vi "HandleObservationSync.vi"(8 "error in (no error)":errorcluster, 11 "S4GUI in":refnum<class "S4GUI.lvclass">) -> (0 "error out":errorcluster, 3 "S4GUI out":refnum<class "S4GUI.lvclass">)   [LabVIEW 2018, in "S4GUI.lvclass"] (continued)
          n1278 = call-dynamic "VerifyAcqIdle.vi"("error in (no error)"=w3499, "S4GUI in"=w3498) -> ("error out"=w3504:errorcluster, "idle"=w3503:bool, "S4GUI out"=w3505:refnum<class "S4GUI.lvclass">)  [unwired: 6 in, 1 out]
          n1279 = disable-structure shown="Enabled" {
            disable-tunnel: w3501 -> [w3508 _]
            disable-tunnel: [w3507 u32 325] -> w3500
            frame Disabled {
              n1280 = Increment(x=w3508) -> (x+1=w3507:u32)
            }
            frame Enabled {
            }
          }
          n1281 = Select(t=w3500, s=w3503, f=w3501) -> (s? t:f=w3502:u32)
          n1282 = Bundle By Name(cluster=w3505, "Obs_state"=w3502) -> (w3506:refnum<class "S4GUI.lvclass">)
        }
        frame 323 {
          n1283 = call-dynamic "Read AcquisitionA.vi"("error in (no error)"=w3572, "S4ACS_GUI in"=w3573) -> ("error out"=w3527:errorcluster, "Acquisition.lvclass"=w3528:refnum<class "Acquisition.lvclass">, "S4ACS_GUI out"=w3575:refnum<class "S4GUI.lvclass">)  [unwired: 7 in]
          n1284 = call-dynamic "Read enabled.vi"("error in (no error)"=w3527, "Server in"=w3528) -> ("error out"=w3526:errorcluster, "enabled"=w3513:bool, "Server out"=w3529:refnum<class "Acquisition.lvclass">)  [unwired: 7 in]
          n1285 = call "Read connection.vi"("error in (no error)"=w3526, "Server in"=w3529) -> ("error out"=w3552:errorcluster, "connection"=w3536:bool, "Server out"=w3553:refnum<class "Acquisition.lvclass">)  [unwired: 7 in]
          n1286 = And(x=w3536, y=w3513) -> (x .and. y?=w3537:bool)
          n1287 = case shown="True" w3537 {
            tunnel: w3553 -> [w3682 w3698]
            tunnel: w3552 -> [w3681 w3697]
            tunnel: [w3682 w3695] -> w3576
            tunnel: [w3681 w3694] -> w3574
            tunnel: [w3678 u32 0 ("New_State")] -> w3542
            tunnel: w3513 -> [w3677 _]
            frame False {
              n1288 = Select(t=u32 1, s=w3677, f=u32 0) -> (s? t:f=w3678:u32)
            }
            frame True {
              n1289 = call-dynamic "Read Channel.vi"("error in (no error)"=w3697, "Acquisition in"=w3698) -> ("error out"=w3690:errorcluster, "Channel.lvclass"=w3689:refnum<class "Channel.lvclass">, "Acquisition out"=w3696:refnum<class "Acquisition.lvclass">)  [unwired: 7 in]
              n1290 = call-dynamic "Read State Machine.vi"("error in (no error)"=w3690, "Device in"=w3689) -> ("error out"=w3691:errorcluster, "State Machine.lvclass"=w3693:refnum<class "State Machine.lvclass">, "Device out"=w3687:refnum<class "Channel.lvclass">)  [unwired: 7 in]
              n1291 = call "Next State.vi"("error in (no error)"=w3691, "New_State"=50, "State Machine in"=w3693) -> ("error out"=w3684:errorcluster, "State Machine out"=w3685:refnum<class "State Machine.lvclass">)  [unwired: 7 in]
              n1292 = call-dynamic "Write State Machine.vi"("error in (no error)"=w3684, "State Machine.lvclass"=w3685, "Device in"=w3687) -> ("error out"=w3686:errorcluster, "Device out"=w3688:refnum<class "Channel.lvclass">)  [unwired: 7 in]
              n1293 = call-dynamic "Write Channel.vi"("error in (no error)"=w3686, "Channel.lvclass"=w3688, "Acquisition in"=w3696) -> ("error out"=w3694:errorcluster, "Acquisition out"=w3695:refnum<class "Acquisition.lvclass">)  [unwired: 7 in]
            }
          }
          n1294 = call-dynamic "Write AcquisitionA.vi"("error in (no error)"=w3574, "Acquisition.lvclass"=w3576, "S4ACS_GUI in"=w3575) -> ("error out"=w3569:errorcluster, "S4ACS_GUI out"=w3570:refnum<class "S4GUI.lvclass">)  [unwired: 7 in]
          n1295 = call "Read AcquisitionB.vi"("error in (no error)"=w3569, "S4ACS_GUI in"=w3570) -> ("error out"=w3523:errorcluster, "Acquisition.lvclass"=w3525:refnum<class "Acquisition.lvclass">, "S4ACS_GUI out"=w3567:refnum<class "S4GUI.lvclass">)  [unwired: 7 in]
          n1296 = call-dynamic "Read enabled.vi"("error in (no error)"=w3523, "Server in"=w3525) -> ("error out"=w3522:errorcluster, "enabled"=w3512:bool, "Server out"=w3524:refnum<class "Acquisition.lvclass">)  [unwired: 7 in]
          n1297 = call "Read connection.vi"("error in (no error)"=w3522, "Server in"=w3524) -> ("error out"=w3550:errorcluster, "connection"=w3534:bool, "Server out"=w3551:refnum<class "Acquisition.lvclass">)  [unwired: 7 in]
          n1298 = And(x=w3534, y=w3512) -> (x .and. y?=w3535:bool)
          n1299 = case shown="True" w3535 {
            tunnel: w3551 -> [w3660 w3676]
            tunnel: w3550 -> [w3659 w3675]
            tunnel: [w3660 w3673] -> w3568
            tunnel: [w3659 w3672] -> w3566
            tunnel: [w3656 u32 0 ("New_State")] -> w3541
            tunnel: w3512 -> [w3655 _]
            frame False {
              n1300 = Select(t=u32 2, s=w3655, f=u32 0) -> (s? t:f=w3656:u32)
            }
            frame True {
              n1301 = call-dynamic "Read Channel.vi"("error in (no error)"=w3675, "Acquisition in"=w3676) -> ("error out"=w3668:errorcluster, "Channel.lvclass"=w3667:refnum<class "Channel.lvclass">, "Acquisition out"=w3674:refnum<class "Acquisition.lvclass">)  [unwired: 7 in]
              n1302 = call-dynamic "Read State Machine.vi"("error in (no error)"=w3668, "Device in"=w3667) -> ("error out"=w3669:errorcluster, "State Machine.lvclass"=w3671:refnum<class "State Machine.lvclass">, "Device out"=w3665:refnum<class "Channel.lvclass">)  [unwired: 7 in]
              n1303 = call "Next State.vi"("error in (no error)"=w3669, "New_State"=50, "State Machine in"=w3671) -> ("error out"=w3662:errorcluster, "State Machine out"=w3663:refnum<class "State Machine.lvclass">)  [unwired: 7 in]
              n1304 = call-dynamic "Write State Machine.vi"("error in (no error)"=w3662, "State Machine.lvclass"=w3663, "Device in"=w3665) -> ("error out"=w3664:errorcluster, "Device out"=w3666:refnum<class "Channel.lvclass">)  [unwired: 7 in]
              n1305 = call-dynamic "Write Channel.vi"("error in (no error)"=w3664, "Channel.lvclass"=w3666, "Acquisition in"=w3674) -> ("error out"=w3672:errorcluster, "Acquisition out"=w3673:refnum<class "Acquisition.lvclass">)  [unwired: 7 in]
            }
          }
          n1306 = call "Write AcquisitionB.vi"("error in (no error)"=w3566, "Acquisition.lvclass"=w3568, "S4ACS_GUI in"=w3567) -> ("error out"=w3562:errorcluster, "S4ACS_GUI out"=w3561:refnum<class "S4GUI.lvclass">)  [unwired: 7 in]
          n1307 = call-dynamic "Read AcquisitionC.vi"("error in (no error)"=w3562, "S4ACS_GUI in"=w3561) -> ("error out"=w3519:errorcluster, "Acquisition.lvclass"=w3521:refnum<class "Acquisition.lvclass">, "S4ACS_GUI out"=w3564:refnum<class "S4GUI.lvclass">)  [unwired: 7 in]
          n1308 = call-dynamic "Read enabled.vi"("error in (no error)"=w3519, "Server in"=w3521) -> ("error out"=w3518:errorcluster, "enabled"=w3511:bool, "Server out"=w3520:refnum<class "Acquisition.lvclass">)  [unwired: 7 in]
          n1309 = call "Read connection.vi"("error in (no error)"=w3518, "Server in"=w3520) -> ("error out"=w3548:errorcluster, "connection"=w3531:bool, "Server out"=w3549:refnum<class "Acquisition.lvclass">)  [unwired: 7 in]
          n1310 = And(x=w3531, y=w3511) -> (x .and. y?=w3533:bool)
          n1311 = case shown="True" w3533 {
            tunnel: [w3637 w3646] -> w3565
            tunnel: [w3638 w3645] -> w3563
            tunnel: w3549 -> [w3638 w3643]
            tunnel: w3548 -> [w3637 w3642]
            tunnel: [w3634 u32 0 ("New_State")] -> w3540
            tunnel: w3511 -> [w3633 _]
            frame False {
              n1312 = Select(t=u32 4, s=w3633, f=u32 0) -> (s? t:f=w3634:u32)
            }
            frame True {
              n1313 = call-dynamic "Read Channel.vi"("error in (no error)"=w3642, "Acquisition in"=w3643) -> ("error out"=w3650:errorcluster, "Channel.lvclass"=w3651:refnum<class "Channel.lvclass">, "Acquisition out"=w3644:refnum<class "Acquisition.lvclass">)  [unwired: 7 in]
              n1314 = call-dynamic "Read State Machine.vi"("error in (no error)"=w3650, "Device in"=w3651) -> ("error out"=w3649:errorcluster, "State Machine.lvclass"=w3647:refnum<class "State Machine.lvclass">, "Device out"=w3653:refnum<class "Channel.lvclass">)  [unwired: 7 in]
              n1315 = call "Next State.vi"("error in (no error)"=w3649, "New_State"=50, "State Machine in"=w3647) -> ("error out"=w3641:errorcluster, "State Machine out"=w3640:refnum<class "State Machine.lvclass">)  [unwired: 7 in]
              n1316 = call-dynamic "Write State Machine.vi"("error in (no error)"=w3641, "State Machine.lvclass"=w3640, "Device in"=w3653) -> ("error out"=w3654:errorcluster, "Device out"=w3652:refnum<class "Channel.lvclass">)  [unwired: 7 in]
              n1317 = call-dynamic "Write Channel.vi"("error in (no error)"=w3654, "Channel.lvclass"=w3652, "Acquisition in"=w3644) -> ("error out"=w3646:errorcluster, "Acquisition out"=w3645:refnum<class "Acquisition.lvclass">)  [unwired: 7 in]
            }
          }
          n1318 = call-dynamic "Write AcquisitionC.vi"("error in (no error)"=w3565, "Acquisition.lvclass"=w3563, "S4ACS_GUI in"=w3564) -> ("error out"=w3559:errorcluster, "S4ACS_GUI out"=w3558:refnum<class "S4GUI.lvclass">)  [unwired: 7 in]
          n1319 = call-dynamic "Read AcquisitionD.vi"("error in (no error)"=w3559, "S4ACS_GUI in"=w3558) -> ("error out"=w3515:errorcluster, "Acquisition.lvclass"=w3517:refnum<class "Acquisition.lvclass">, "S4ACS_GUI out"=w3557:refnum<class "S4GUI.lvclass">)  [unwired: 7 in]
          n1320 = call-dynamic "Read enabled.vi"("error in (no error)"=w3515, "Server in"=w3517) -> ("error out"=w3514:errorcluster, "enabled"=w3510:bool, "Server out"=w3516:refnum<class "Acquisition.lvclass">)  [unwired: 7 in]
          n1321 = call "Read connection.vi"("error in (no error)"=w3514, "Server in"=w3516) -> ("error out"=w3546:errorcluster, "connection"=w3530:bool, "Server out"=w3547:refnum<class "Acquisition.lvclass">)  [unwired: 7 in]
          n1322 = And(x=w3530, y=w3510) -> (x .and. y?=w3532:bool)
          n1323 = case shown="True" w3532 {
            tunnel: w3546 -> [w3615 w3632]
            tunnel: [w3615 w3631] -> w3560
            tunnel: w3547 -> [w3616 w3622]
            tunnel: [w3616 w3620] -> w3556
            tunnel: [w3612 u32 0 ("New_State")] -> w3539
            tunnel: w3510 -> [w3611 _]
            frame False {
              n1324 = Select(t=u32 8, s=w3611, f=u32 0) -> (s? t:f=w3612:u32)
            }
            frame True {
              n1325 = call-dynamic "Read Channel.vi"("error in (no error)"=w3632, "Acquisition in"=w3622) -> ("error out"=w3627:errorcluster, "Channel.lvclass"=w3626:refnum<class "Channel.lvclass">, "Acquisition out"=w3621:refnum<class "Acquisition.lvclass">)  [unwired: 7 in]
              n1326 = call-dynamic "Read State Machine.vi"("error in (no error)"=w3627, "Device in"=w3626) -> ("error out"=w3628:errorcluster, "State Machine.lvclass"=w3630:refnum<class "State Machine.lvclass">, "Device out"=w3624:refnum<class "Channel.lvclass">)  [unwired: 7 in]
              n1327 = call "Next State.vi"("error in (no error)"=w3628, "New_State"=50, "State Machine in"=w3630) -> ("error out"=w3618:errorcluster, "State Machine out"=w3619:refnum<class "State Machine.lvclass">)  [unwired: 7 in]
              n1328 = call-dynamic "Write State Machine.vi"("error in (no error)"=w3618, "State Machine.lvclass"=w3619, "Device in"=w3624) -> ("error out"=w3623:errorcluster, "Device out"=w3625:refnum<class "Channel.lvclass">)  [unwired: 7 in]
              n1329 = call-dynamic "Write Channel.vi"("error in (no error)"=w3623, "Channel.lvclass"=w3625, "Acquisition in"=w3621) -> ("error out"=w3631:errorcluster, "Acquisition out"=w3620:refnum<class "Acquisition.lvclass">)  [unwired: 7 in]
            }
          }
          n1330 = call-dynamic "Write AcquisitionD.vi"("error in (no error)"=w3560, "Acquisition.lvclass"=w3556, "S4ACS_GUI in"=w3557) -> ("error out"=w3555:errorcluster, "S4ACS_GUI out"=w3554:refnum<class "S4GUI.lvclass">)  [unwired: 7 in]
          n1331 = Compound Arithmetic op=ADD(w3542, w3541, w3540, w3539) -> (w3543:u32)
          n1332 = case shown="0, Default" w3543 {
            tunnel: w3538 -> [w3580 _ _ _ _ _ _ _ _ _ _ _ _ _ _ _]
            tunnel: [w3579 u32 1 ("Obs_state") u32 1 ("Obs_state") u32 1 ("Obs_state") u32 1 ("Obs_state") u32 1 ("Obs_state") u32 1 ("Obs_state") u32 1 ("Obs_state") u32 1 ("Obs_state") u32 1 ("Obs_state") u32 1 ("Obs_state") u32 1 ("Obs_state") u32 1 ("Obs_state") u32 1 ("Obs_state") u32 1 ("Obs_state") u32 1 ("Obs_state")] -> w3544
            tunnel: ["" ("Error Msg") "ERROR: Lost channel 1 connection... - HandleObservationSync.vi state 323" ("Error Msg") "ERROR: Lost channel 2 connection...- HandleObservationSync.vi state 323" ("Error Msg") "ERROR: Lost channels 1 and 2 connection...- HandleObservationSync.vi state 323" ("Error Msg") "ERROR: Lost channel 3 connection...- HandleObservationSync.vi state 323" ("Error Msg") "ERROR: Lost channels 1 and  3 connection...- HandleObservationSync.vi state 323" ("Error Msg") "ERROR:  Lost channels 2 and  3 connection...- HandleObservationSync.vi state 323" ("Error Msg") "ERROR:  Lost channels 1, 2 and  3 connection...- HandleObservationSync.vi state 323" ("Error Msg") "ERROR: Lost channel 4 connection...- HandleObservationSync.vi state 323" ("Error Msg") "ERROR:  Lost channels 1 and 4 connection...- HandleObservationSync.vi state 323" ("Error Msg") "ERROR:  Lost channels 2 and 4 connection...- HandleObservationSync.vi state 323" ("Error Msg") "ERROR: Lost channels 1, 2 and 4 connection...- HandleObservationSync.vi state 323" ("Error Msg") "ERROR: Lost channels 3 and 4 connection...- HandleObservationSync.vi state 323" ("Error Msg") "ERROR: Lost channels 1, 3 and 4 connection...- HandleObservationSync.vi state 323" ("Error Msg") "ERROR: Lost channels 2, 3 and 4 connection...- HandleObservationSync.vi state 323" ("Error Msg") "ERROR: Lost channels 1, 2, 3 and 4 connection...- HandleObservationSync.vi state 323" ("Error Msg")] -> w3545
            frame 0, Default {
              n1333 = Increment(x=w3580) -> (x+1=w3579:u32)
              n1334 = Tick Count (ms)() -> (millisecond timer value=w3577:u32)
              n1335 = local write "time1"(w3577) -> ()
            }
            frame 1 {
            }
            frame 2 {
            }
            frame 3 {
            }
            frame 4 {
            }
            frame 5 {
            }
            frame 6 {
            }
            frame 7 {
            }
            frame 8 {
            }
            frame 9 {
            }
            frame 10 {
            }
            frame 11 {
            }
            frame 12 {
            }
            frame 13 {
            }
            frame 14 {
            }
            frame 15 {
            }
          }
          n1336 = Bundle By Name(cluster=w3554, "Obs_state"=w3544, "Error Msg"=w3545) -> (w3571:refnum<class "S4GUI.lvclass">)
        }
        frame 324 {
          # "Espera terminar a execução do comando atual \nantes de ir ao proximo passo da Observação."
          n1337 = call-dynamic "Read AcquisitionA.vi"("error in (no error)"=w3752, "S4ACS_GUI in"=w3753) -> ("error out"=w3734:errorcluster, "Acquisition.lvclass"=w3735:refnum<class "Acquisition.lvclass">, "S4ACS_GUI out"=w3755:refnum<class "S4GUI.lvclass">)  [unwired: 7 in]
          n1338 = call "Read connection.vi"("error in (no error)"=w3734, "Server in"=w3735) -> ("error out"=w3733:errorcluster, "connection"=w3732:bool, "Server out"=w3731:refnum<class "Acquisition.lvclass">)  [unwired: 7 in]
          n1339 = case shown="True" w3732 {
            tunnel: w3733 -> [w3864 w3885]
            tunnel: [w3865 w3883] -> w3756
            tunnel: [w3864 w3882] -> w3754
            tunnel: [TRUE w3871] -> w3713
            tunnel: w3731 -> [w3865 w3874]
            tunnel: [FALSE w3866] -> w3711
            frame False {
            }
            frame True {
              n1340 = call-dynamic "Read Channel.vi"("error in (no error)"=w3885, "Acquisition in"=w3874) -> ("error out"=w3868:errorcluster, "Channel.lvclass"=w3870:refnum<class "Channel.lvclass">, "Acquisition out"=w3884:refnum<class "Acquisition.lvclass">)  [unwired: 7 in]
              n1341 = call-dynamic "Read wait_expose.vi"("error in (no error)"=w3868, "Channel in"=w3870) -> ("error out"=w3867:errorcluster, "wait_expose"=w3866:bool, "Channel out"=w3869:refnum<class "Channel.lvclass">)  [unwired: 7 in]
              n1342 = call-dynamic "Read State Machine.vi"("error in (no error)"=w3867, "Device in"=w3869) -> ("error out"=w3876:errorcluster, "State Machine.lvclass"=w3878:refnum<class "State Machine.lvclass">, "Device out"=w3880:refnum<class "Channel.lvclass">)  [unwired: 7 in]
              n1343 = call-dynamic "Read State.vi"("error in (no error)"=w3876, "State Machine in"=w3878) -> ("error out"=w3875:errorcluster, "State"=w3872:i32, "State Machine out"=w3877:refnum<class "State Machine.lvclass">)  [unwired: 7 in]
              n1344 = Greater?(x=w3872, y=53 ("x")) -> (0:w3871:bool)
              n1345 = call-dynamic "Write State Machine.vi"("error in (no error)"=w3875, "State Machine.lvclass"=w3877, "Device in"=w3880) -> ("error out"=w3879:errorcluster, "Device out"=w3881:refnum<class "Channel.lvclass">)  [unwired: 7 in]
              n1346 = call-dynamic "Write Channel.vi"("error in (no error)"=w3879, "Channel.lvclass"=w3881, "Acquisition in"=w3884) -> ("error out"=w3882:errorcluster, "Acquisition out"=w3883:refnum<class "Acquisition.lvclass">)  [unwired: 7 in]
            }
          }
          n1347 = call-dynamic "Write AcquisitionA.vi"("error in (no error)"=w3754, "Acquisition.lvclass"=w3756, "S4ACS_GUI in"=w3755) -> ("error out"=w3749:errorcluster, "S4ACS_GUI out"=w3748:refnum<class "S4GUI.lvclass">)  [unwired: 7 in]
          n1348 = call "Read AcquisitionB.vi"("error in (no error)"=w3749, "S4ACS_GUI in"=w3748) -> ("error out"=w3726:errorcluster, "Acquisition.lvclass"=w3730:refnum<class "Acquisition.lvclass">, "S4ACS_GUI out"=w3750:refnum<class "S4GUI.lvclass">)  [unwired: 7 in]
          n1349 = call "Read connection.vi"("error in (no error)"=w3726, "Server in"=w3730) -> ("error out"=w3727:errorcluster, "connection"=w3728:bool, "Server out"=w3729:refnum<class "Acquisition.lvclass">)  [unwired: 7 in]
          n1350 = case shown="True" w3728 {
            tunnel: w3727 -> [w3840 w3853]
            tunnel: w3729 -> [w3841 w3852]
            tunnel: [TRUE w3847] -> w3715
            tunnel: [w3840 w3851] -> w3747
            tunnel: [w3841 w3850] -> w3746
            tunnel: [FALSE w3842] -> w3710
            frame False {
            }
            frame True {
              n1351 = call-dynamic "Read Channel.vi"("error in (no error)"=w3853, "Acquisition in"=w3852) -> ("error out"=w3844:errorcluster, "Channel.lvclass"=w3846:refnum<class "Channel.lvclass">, "Acquisition out"=w3854:refnum<class "Acquisition.lvclass">)  [unwired: 7 in]
              n1352 = call-dynamic "Read wait_expose.vi"("error in (no error)"=w3844, "Channel in"=w3846) -> ("error out"=w3843:errorcluster, "wait_expose"=w3842:bool, "Channel out"=w3845:refnum<class "Channel.lvclass">)  [unwired: 7 in]
              n1353 = call-dynamic "Read State Machine.vi"("error in (no error)"=w3843, "Device in"=w3845) -> ("error out"=w3860:errorcluster, "State Machine.lvclass"=w3858:refnum<class "State Machine.lvclass">, "Device out"=w3856:refnum<class "Channel.lvclass">)  [unwired: 7 in]
              n1354 = call-dynamic "Read State.vi"("error in (no error)"=w3860, "State Machine in"=w3858) -> ("error out"=w3861:errorcluster, "State"=w3849:i32, "State Machine out"=w3859:refnum<class "State Machine.lvclass">)  [unwired: 7 in]
              n1355 = Greater?(x=w3849, y=53 ("x")) -> (0:w3847:bool)
              n1356 = call-dynamic "Write State Machine.vi"("error in (no error)"=w3861, "State Machine.lvclass"=w3859, "Device in"=w3856) -> ("error out"=w3857:errorcluster, "Device out"=w3855:refnum<class "Channel.lvclass">)  [unwired: 7 in]
              n1357 = call-dynamic "Write Channel.vi"("error in (no error)"=w3857, "Channel.lvclass"=w3855, "Acquisition in"=w3854) -> ("error out"=w3851:errorcluster, "Acquisition out"=w3850:refnum<class "Acquisition.lvclass">)  [unwired: 7 in]
            }
          }
          n1358 = call "Write AcquisitionB.vi"("error in (no error)"=w3747, "Acquisition.lvclass"=w3746, "S4ACS_GUI in"=w3750) -> ("error out"=w3739:errorcluster, "S4ACS_GUI out"=w3738:refnum<class "S4GUI.lvclass">)  [unwired: 7 in]
          n1359 = call-dynamic "Read AcquisitionC.vi"("error in (no error)"=w3739, "S4ACS_GUI in"=w3738) -> ("error out"=w3722:errorcluster, "Acquisition.lvclass"=w3725:refnum<class "Acquisition.lvclass">, "S4ACS_GUI out"=w3741:refnum<class "S4GUI.lvclass">)  [unwired: 7 in]
          n1360 = call "Read connection.vi"("error in (no error)"=w3722, "Server in"=w3725) -> ("error out"=w3721:errorcluster, "connection"=w3723:bool, "Server out"=w3724:refnum<class "Acquisition.lvclass">)  [unwired: 7 in]
          n1361 = case shown="True" w3723 {
            tunnel: [w3816 w3830] -> w3742
            tunnel: [w3817 w3829] -> w3740
            tunnel: w3721 -> [w3816 w3826]
            tunnel: w3724 -> [w3817 w3827]
            tunnel: [TRUE w3823] -> w3714
            tunnel: [FALSE w3818] -> w3709
            frame False {
            }
            frame True {
              n1362 = call-dynamic "Read Channel.vi"("error in (no error)"=w3826, "Acquisition in"=w3827) -> ("error out"=w3820:errorcluster, "Channel.lvclass"=w3822:refnum<class "Channel.lvclass">, "Acquisition out"=w3828:refnum<class "Acquisition.lvclass">)  [unwired: 7 in]
              n1363 = call-dynamic "Read wait_expose.vi"("error in (no error)"=w3820, "Channel in"=w3822) -> ("error out"=w3819:errorcluster, "wait_expose"=w3818:bool, "Channel out"=w3821:refnum<class "Channel.lvclass">)  [unwired: 7 in]
              n1364 = call-dynamic "Read State Machine.vi"("error in (no error)"=w3819, "Device in"=w3821) -> ("error out"=w3836:errorcluster, "State Machine.lvclass"=w3834:refnum<class "State Machine.lvclass">, "Device out"=w3832:refnum<class "Channel.lvclass">)  [unwired: 7 in]
              n1365 = call-dynamic "Read State.vi"("error in (no error)"=w3836, "State Machine in"=w3834) -> ("error out"=w3837:errorcluster, "State"=w3824:i32, "State Machine out"=w3835:refnum<class "State Machine.lvclass">)  [unwired: 7 in]
              n1366 = Greater?(x=w3824, y=53 ("x")) -> (0:w3823:bool)
              n1367 = call-dynamic "Write State Machine.vi"("error in (no error)"=w3837, "State Machine.lvclass"=w3835, "Device in"=w3832) -> ("error out"=w3833:errorcluster, "Device out"=w3831:refnum<class "Channel.lvclass">)  [unwired: 7 in]
              n1368 = call-dynamic "Write Channel.vi"("error in (no error)"=w3833, "Channel.lvclass"=w3831, "Acquisition in"=w3828) -> ("error out"=w3830:errorcluster, "Acquisition out"=w3829:refnum<class "Acquisition.lvclass">)  [unwired: 7 in]
            }
          }
          n1369 = call-dynamic "Write AcquisitionC.vi"("error in (no error)"=w3742, "Acquisition.lvclass"=w3740, "S4ACS_GUI in"=w3741) -> ("error out"=w3736:errorcluster, "S4ACS_GUI out"=w3737:refnum<class "S4GUI.lvclass">)  [unwired: 7 in]
          n1370 = call-dynamic "Read AcquisitionD.vi"("error in (no error)"=w3736, "S4ACS_GUI in"=w3737) -> ("error out"=w3717:errorcluster, "Acquisition.lvclass"=w3720:refnum<class "Acquisition.lvclass">, "S4ACS_GUI out"=w3743:refnum<class "S4GUI.lvclass">)  [unwired: 7 in]
          n1371 = call "Read connection.vi"("error in (no error)"=w3717, "Server in"=w3720) -> ("error out"=w3716:errorcluster, "connection"=w3718:bool, "Server out"=w3719:refnum<class "Acquisition.lvclass">)  [unwired: 7 in]
          n1372 = case shown="True" w3718 {
            tunnel: [w3793 w3813] -> w3745
            tunnel: [w3792 w3812] -> w3744
            tunnel: w3719 -> [w3793 w3811]
            tunnel: w3716 -> [w3792 w3810]
            tunnel: [TRUE w3799] -> w3712
            tunnel: [FALSE w3794] -> w3708
            frame False {
            }
            frame True {
              n1373 = call-dynamic "Read Channel.vi"("error in (no error)"=w3810, "Acquisition in"=w3811) -> ("error out"=w3796:errorcluster, "Channel.lvclass"=w3798:refnum<class "Channel.lvclass">, "Acquisition out"=w3809:refnum<class "Acquisition.lvclass">)  [unwired: 7 in]
              n1374 = call-dynamic "Read wait_expose.vi"("error in (no error)"=w3796, "Channel in"=w3798) -> ("error out"=w3795:errorcluster, "wait_expose"=w3794:bool, "Channel out"=w3797:refnum<class "Channel.lvclass">)  [unwired: 7 in]
              n1375 = call-dynamic "Read State Machine.vi"("error in (no error)"=w3795, "Device in"=w3797) -> ("error out"=w3803:errorcluster, "State Machine.lvclass"=w3805:refnum<class "State Machine.lvclass">, "Device out"=w3807:refnum<class "Channel.lvclass">)  [unwired: 7 in]
              n1376 = call-dynamic "Read State.vi"("error in (no error)"=w3803, "State Machine in"=w3805) -> ("error out"=w3802:errorcluster, "State"=w3800:i32, "State Machine out"=w3804:refnum<class "State Machine.lvclass">)  [unwired: 7 in]
              n1377 = Greater?(x=w3800, y=53 ("x")) -> (0:w3799:bool)
              n1378 = call-dynamic "Write State Machine.vi"("error in (no error)"=w3802, "State Machine.lvclass"=w3804, "Device in"=w3807) -> ("error out"=w3806:errorcluster, "Device out"=w3808:refnum<class "Channel.lvclass">)  [unwired: 7 in]
              n1379 = call-dynamic "Write Channel.vi"("error in (no error)"=w3806, "Channel.lvclass"=w3808, "Acquisition in"=w3809) -> ("error out"=w3812:errorcluster, "Acquisition out"=w3813:refnum<class "Acquisition.lvclass">)  [unwired: 7 in]
            }
          }
          n1380 = call-dynamic "Write AcquisitionD.vi"("error in (no error)"=w3744, "Acquisition.lvclass"=w3745, "S4ACS_GUI in"=w3743) -> ("error out"=w3700:errorcluster, "S4ACS_GUI out"=w3703:refnum<class "S4GUI.lvclass">)  [unwired: 7 in]
          n1381 = Compound Arithmetic op=AND(w3713, w3715, w3714, w3712) -> (w3707:bool)
          n1382 = Compound Arithmetic op=OR(w3711, w3710, w3709, w3708) -> (w3705:bool)
          n1383 = call-dynamic "VerifErrors.vi"("error in (no error)"=w3700, "S4GUI in"=w3703) -> ("error out"=w3699:errorcluster, "Error value"=w3702:u32, "S4GUI out"=w3701:refnum<class "S4GUI.lvclass">)  [unwired: 7 in]
          n1384 = case shown="False" w3707 {
            tunnel: w3701 -> [w3759 w3789]
            tunnel: [w3765 w3788] -> w3704
            tunnel: w3706 -> [_ w3787]
            tunnel: w3705 -> [_ w3783]
            tunnel: w3702 -> [w3757 _]
            frame False {
              # "Aguardando iniciar exposição por 5s"
              n1385 = Tick Count (ms)() -> (millisecond timer value=w3764:u32)
              n1386 = local read "time1"() -> (w3758:u32)
              n1387 = Subtract(x=w3764, y=w3758) -> (x-y=w3761:u32)
              n1388 = To Double Precision Float(number=w3761) -> (double precision float=w3763:dbl)
              n1389 = Less?(x=5000.0 ("y"), y=w3763) -> (x < y?=w3762:bool)
              n1390 = case shown="False" w3762 {
                tunnel: w3759 -> [w3768 w3781]
                tunnel: [w3766 w3780] -> w3765
                tunnel: w3757 -> [w3767 _]
                frame False {
                  n1391 = case shown="1..15" w3767 {
                    selector: w3767 -> [_ w3776]
                    tunnel: [w3769 w3771] -> w3766
                    tunnel: w3768 -> [w3769 w3777]
                    frame 0, Default {
                    }
                    frame 1..15 {
                      n1392 = Number To Decimal String(number=w3776) -> (decimal integer string=w3773:string)  [unwired: 1 in]
                      n1393 = Concatenate Strings("CHANNEL ERROR <", w3773, ">: Error flag TRUE - see ACS panel.  HandleObservationSync.vi - state 324.") -> (w3775:string)
                      n1394 = Bundle By Name(cluster=w3777, "Obs_state"=u32 1, "Error Msg"=w3775) -> (w3771:refnum<class "S4GUI.lvclass">)
                    }
                  }
                }
                frame True {
                  n1395 = Bundle By Name(cluster=w3781, "Obs_state"=u32 1, "Error Msg"="ERROR: Acquisition Timeout. HandleObservationSync.vi - state 324.") -> (w3780:refnum<class "S4GUI.lvclass">)
                }
              }
            }
            frame True {
              # "327: Verifica incremento de ciclo."
              # "Iniciou aquisição..."
              n1396 = Increment(x=w3787) -> (x+1=w3784:u32)
              n1397 = Select(t=u32 327, s=w3783, f=w3784) -> (s? t:f=w3782:u32)
              n1398 = Tick Count (ms)() -> (millisecond timer value=w3786:u32)
              n1399 = Bundle By Name(cluster=w3789, "Obs_state"=w3782) -> (w3788:refnum<class "S4GUI.lvclass">)
              n1400 = local write "time307"(w3786) -> ()
            }
          }
          n1401 = Bundle By Name(cluster=w3704, "mode EXPOSE"=w3705) -> (w3751:refnum<class "S4GUI.lvclass">)
        }
        frame 325 {
          n1402 = Unbundle By Name(w3895) -> ("mode EXPOSE"=w3894:bool)
          n1403 = case shown="True" w3894 {
            tunnel: w3895 -> [w3948 w4015]
            tunnel: w3900 -> [w3947 w4014]
            tunnel: [w3946 w4012] -> w3899
            tunnel: [w3945 w4013] -> w3898
            tunnel: [w3944 w4011] -> w3888
            tunnel: w3896 -> [w3936 w4011]
            tunnel: [w3935 w3976] -> w3893
            tunnel: [w3935 w3975] -> w3892
            tunnel: [w3935 w3974] -> w3891
            tunnel: [w3935 w3973] -> w3890
            frame False {
              w3935 = 0
              n1404 = call-dynamic "Read Sync Box.lvclass.vi"("error in (no error)"=w3947, "SPARC4_AC in"=w3948) -> ("error out"=w3941:errorcluster, "Sync Box.lvclass"=w3943:refnum<class "Sync Box.lvclass">, "SPARC4_AC out"=w3938:refnum<class "S4GUI.lvclass">)  [unwired: 7 in]
              n1405 = call "Read connection.vi"("error in (no error)"=w3941, "Server in"=w3943) -> ("error out"=w3940:errorcluster, "connection"=w3939:bool, "Server out"=w3942:refnum<class "Sync Box.lvclass">)  [unwired: 7 in]
              n1406 = case shown="True" w3939 {
                tunnel: w3940 -> [w3954 w3972]
                tunnel: [w3955 w3970] -> w3950
                tunnel: [w3954 w3957] -> w3949
                tunnel: w3936 -> [w3951 w3956]
                tunnel: [w3953 w3956] -> w3944
                tunnel: w3942 -> [w3955 w3961]
                tunnel: w3938 -> [w3952 w3958]
                tunnel: [w3952 w3958] -> w3937
                frame False {
                  n1407 = Increment(x=w3951) -> (x+1=w3953:u32)
                }
                frame True {
                  # "Envia comando FIRE para o SyncBox"
                  n1408 = call-dynamic "Read Trigger.lvclass.vi"("error in (no error)"=w3972, "Sync Box in"=w3961) -> ("error out"=w3966:errorcluster, "Trigger.lvclass"=w3965:refnum<class "Trigger.lvclass">, "Sync Box out"=w3971:refnum<class "Sync Box.lvclass">)  [unwired: 7 in]
                  n1409 = call-dynamic "Read State Machine.vi"("error in (no error)"=w3966, "Device in"=w3965) -> ("error out"=w3967:errorcluster, "State Machine.lvclass"=w3969:refnum<class "State Machine.lvclass">, "Device out"=w3963:refnum<class "Trigger.lvclass">)  [unwired: 7 in]
                  n1410 = call "Next State.vi"("error in (no error)"=w3967, "New_State"=40, "State Machine in"=w3969) -> ("error out"=w3959:errorcluster, "State Machine out"=w3960:refnum<class "State Machine.lvclass">)  [unwired: 7 in]
                  n1411 = call-dynamic "Write State Machine.vi"("error in (no error)"=w3959, "State Machine.lvclass"=w3960, "Device in"=w3963) -> ("error out"=w3962:errorcluster, "Device out"=w3964:refnum<class "Trigger.lvclass">)  [unwired: 7 in]
                  n1412 = call-dynamic "Write Trigger.lvclass.vi"("error in (no error)"=w3962, "Trigger.lvclass"=w3964, "Sync Box in"=w3971) -> ("error out"=w3957:errorcluster, "Sync Box out"=w3970:refnum<class "Sync Box.lvclass">)  [unwired: 7 in]
                }
              }
              n1413 = call-dynamic "Write Sync Box.lvclass.vi"("error in (no error)"=w3949, "Sync Box.lvclass"=w3950, "SPARC4_AC in"=w3937) -> ("error out"=w3946:errorcluster, "SPARC4_AC out"=w3945:refnum<class "S4GUI.lvclass">)  [unwired: 7 in]
            }
            frame True {
              # "Envia comando EXPOSE para os canais ativos"
              n1414 = call-dynamic "Read AcquisitionA.vi"("error in (no error)"=w4014, "S4ACS_GUI in"=w4015) -> ("error out"=w4008:errorcluster, "Acquisition.lvclass"=w4010:refnum<class "Acquisition.lvclass">, "S4ACS_GUI out"=w4034:refnum<class "S4GUI.lvclass">)  [unwired: 7 in]
              n1415 = call-dynamic "Read enabled.vi"("error in (no error)"=w4008, "Server in"=w4010) -> ("error out"=w4007:errorcluster, "enabled"=w3980:bool, "Server out"=w4009:refnum<class "Acquisition.lvclass">)  [unwired: 7 in]
              n1416 = call "Read connection.vi"("error in (no error)"=w4007, "Server in"=w4009) -> ("error out"=w4016:errorcluster, "connection"=w4005:bool, "Server out"=w4017:refnum<class "Acquisition.lvclass">)  [unwired: 7 in]
              n1417 = And(x=w4005, y=w3980) -> (x .and. y?=w4006:bool)
              n1418 = case shown="False" w4006 {
                tunnel: w4017 -> [w4107 w4123]
                tunnel: w4016 -> [w4106 w4122]
                tunnel: [w4107 w4120] -> w4035
                tunnel: [w4106 w4119] -> w4033
                tunnel: [w4102 0] -> w3976
                tunnel: w3980 -> [w4103 _]
                frame False {
                  n1419 = Select(t=1, s=w4103, f=0) -> (s? t:f=w4102:i32)
                }
                frame True {
                  n1420 = call-dynamic "Read Channel.vi"("error in (no error)"=w4122, "Acquisition in"=w4123) -> ("error out"=w4115:errorcluster, "Channel.lvclass"=w4114:refnum<class "Channel.lvclass">, "Acquisition out"=w4121:refnum<class "Acquisition.lvclass">)  [unwired: 7 in]
                  n1421 = call-dynamic "Read State Machine.vi"("error in (no error)"=w4115, "Device in"=w4114) -> ("error out"=w4116:errorcluster, "State Machine.lvclass"=w4118:refnum<class "State Machine.lvclass">, "Device out"=w4112:refnum<class "Channel.lvclass">)  [unwired: 7 in]
                  n1422 = call "Next State.vi"("error in (no error)"=w4116, "New_State"=50, "State Machine in"=w4118) -> ("error out"=w4109:errorcluster, "State Machine out"=w4110:refnum<class "State Machine.lvclass">)  [unwired: 7 in]
                  n1423 = call-dynamic "Write State Machine.vi"("error in (no error)"=w4109, "State Machine.lvclass"=w4110, "Device in"=w4112) -> ("error out"=w4111:errorcluster, "Device out"=w4113:refnum<class "Channel.lvclass">)  [unwired: 7 in]
                  n1424 = call-dynamic "Write Channel.vi"("error in (no error)"=w4111, "Channel.lvclass"=w4113, "Acquisition in"=w4121) -> ("error out"=w4119:errorcluster, "Acquisition out"=w4120:refnum<class "Acquisition.lvclass">)  [unwired: 7 in]
                }
              }
              n1425 = call-dynamic "Write AcquisitionA.vi"("error in (no error)"=w4033, "Acquisition.lvclass"=w4035, "S4ACS_GUI in"=w4034) -> ("error out"=w4031:errorcluster, "S4ACS_GUI out"=w4032:refnum<class "S4GUI.lvclass">)  [unwired: 7 in]
              n1426 = call "Read AcquisitionB.vi"("error in (no error)"=w4031, "S4ACS_GUI in"=w4032) -> ("error out"=w3999:errorcluster, "Acquisition.lvclass"=w4001:refnum<class "Acquisition.lvclass">, "S4ACS_GUI out"=w4029:refnum<class "S4GUI.lvclass">)  [unwired: 7 in]
              n1427 = call-dynamic "Read enabled.vi"("error in (no error)"=w3999, "Server in"=w4001) -> ("error out"=w4003:errorcluster, "enabled"=w3979:bool, "Server out"=w4004:refnum<class "Acquisition.lvclass">)  [unwired: 7 in]
              n1428 = call "Read connection.vi"("error in (no error)"=w4003, "Server in"=w4004) -> ("error out"=w3998:errorcluster, "connection"=w4002:bool, "Server out"=w4000:refnum<class "Acquisition.lvclass">)  [unwired: 7 in]
              n1429 = And(x=w4002, y=w3979) -> (x .and. y?=w3997:bool)
              n1430 = case shown="True" w3997 {
                tunnel: w4000 -> [w4085 w4101]
                tunnel: w3998 -> [w4084 w4100]
                tunnel: [w4085 w4098] -> w4030
                tunnel: [w4084 w4097] -> w4028
                tunnel: [w4081 0] -> w3975
                tunnel: w3979 -> [w4080 _]
                frame False {
                  n1431 = Select(t=2, s=w4080, f=0) -> (s? t:f=w4081:i32)
                }
                frame True {
                  n1432 = call-dynamic "Read Channel.vi"("error in (no error)"=w4100, "Acquisition in"=w4101) -> ("error out"=w4093:errorcluster, "Channel.lvclass"=w4092:refnum<class "Channel.lvclass">, "Acquisition out"=w4099:refnum<class "Acquisition.lvclass">)  [unwired: 7 in]
                  n1433 = call-dynamic "Read State Machine.vi"("error in (no error)"=w4093, "Device in"=w4092) -> ("error out"=w4094:errorcluster, "State Machine.lvclass"=w4096:refnum<class "State Machine.lvclass">, "Device out"=w4090:refnum<class "Channel.lvclass">)  [unwired: 7 in]
                  n1434 = call "Next State.vi"("error in (no error)"=w4094, "New_State"=50, "State Machine in"=w4096) -> ("error out"=w4087:errorcluster, "State Machine out"=w4088:refnum<class "State Machine.lvclass">)  [unwired: 7 in]
                  n1435 = call-dynamic "Write State Machine.vi"("error in (no error)"=w4087, "State Machine.lvclass"=w4088, "Device in"=w4090) -> ("error out"=w4089:errorcluster, "Device out"=w4091:refnum<class "Channel.lvclass">)  [unwired: 7 in]
                  n1436 = call-dynamic "Write Channel.vi"("error in (no error)"=w4089, "Channel.lvclass"=w4091, "Acquisition in"=w4099) -> ("error out"=w4097:errorcluster, "Acquisition out"=w4098:refnum<class "Acquisition.lvclass">)  [unwired: 7 in]
                }
              }
              n1437 = call "Write AcquisitionB.vi"("error in (no error)"=w4028, "Acquisition.lvclass"=w4030, "S4ACS_GUI in"=w4029) -> ("error out"=w4024:errorcluster, "S4ACS_GUI out"=w4023:refnum<class "S4GUI.lvclass">)  [unwired: 7 in]
              n1438 = call-dynamic "Read AcquisitionC.vi"("error in (no error)"=w4024, "S4ACS_GUI in"=w4023) -> ("error out"=w3990:errorcluster, "Acquisition.lvclass"=w3991:refnum<class "Acquisition.lvclass">, "S4ACS_GUI out"=w4026:refnum<class "S4GUI.lvclass">)  [unwired: 7 in]
              n1439 = call-dynamic "Read enabled.vi"("error in (no error)"=w3990, "Server in"=w3991) -> ("error out"=w3995:errorcluster, "enabled"=w3978:bool, "Server out"=w3996:refnum<class "Acquisition.lvclass">)  [unwired: 7 in]
              n1440 = call "Read connection.vi"("error in (no error)"=w3995, "Server in"=w3996) -> ("error out"=w3992:errorcluster, "connection"=w3994:bool, "Server out"=w3993:refnum<class "Acquisition.lvclass">)  [unwired: 7 in]
              n1441 = And(x=w3994, y=w3978) -> (x .and. y?=w3989:bool)
              n1442 = case shown="False" w3989 {
                tunnel: [w4062 w4071] -> w4027
                tunnel: [w4063 w4070] -> w4025
                tunnel: w3993 -> [w4063 w4068]
                tunnel: w3992 -> [w4062 w4067]
                tunnel: [w4058 0] -> w3974
                tunnel: w3978 -> [w4059 _]
                frame False {
                  n1443 = Select(t=4, s=w4059, f=0) -> (s? t:f=w4058:i32)
                }
                frame True {
                  n1444 = call-dynamic "Read Channel.vi"("error in (no error)"=w4067, "Acquisition in"=w4068) -> ("error out"=w4075:errorcluster, "Channel.lvclass"=w4076:refnum<class "Channel.lvclass">, "Acquisition out"=w4069:refnum<class "Acquisition.lvclass">)  [unwired: 7 in]
                  n1445 = call-dynamic "Read State Machine.vi"("error in (no error)"=w4075, "Device in"=w4076) -> ("error out"=w4074:errorcluster, "State Machine.lvclass"=w4072:refnum<class "State Machine.lvclass">, "Device out"=w4078:refnum<class "Channel.lvclass">)  [unwired: 7 in]
                  n1446 = call "Next State.vi"("error in (no error)"=w4074, "New_State"=50, "State Machine in"=w4072) -> ("error out"=w4066:errorcluster, "State Machine out"=w4065:refnum<class "State Machine.lvclass">)  [unwired: 7 in]
                  n1447 = call-dynamic "Write State Machine.vi"("error in (no error)"=w4066, "State Machine.lvclass"=w4065, "Device in"=w4078) -> ("error out"=w4079:errorcluster, "Device out"=w4077:refnum<class "Channel.lvclass">)  [unwired: 7 in]
                  n1448 = call-dynamic "Write Channel.vi"("error in (no error)"=w4079, "Channel.lvclass"=w4077, "Acquisition in"=w4069) -> ("error out"=w4071:errorcluster, "Acquisition out"=w4070:refnum<class "Acquisition.lvclass">)  [unwired: 7 in]
                }
              }
              n1449 = call-dynamic "Write AcquisitionC.vi"("error in (no error)"=w4027, "Acquisition.lvclass"=w4025, "S4ACS_GUI in"=w4026) -> ("error out"=w4021:errorcluster, "S4ACS_GUI out"=w4020:refnum<class "S4GUI.lvclass">)  [unwired: 7 in]
              n1450 = call-dynamic "Read AcquisitionD.vi"("error in (no error)"=w4021, "S4ACS_GUI in"=w4020) -> ("error out"=w3982:errorcluster, "Acquisition.lvclass"=w3983:refnum<class "Acquisition.lvclass">, "S4ACS_GUI out"=w4019:refnum<class "S4GUI.lvclass">)  [unwired: 7 in]
              n1451 = call-dynamic "Read enabled.vi"("error in (no error)"=w3982, "Server in"=w3983) -> ("error out"=w3987:errorcluster, "enabled"=w3977:bool, "Server out"=w3988:refnum<class "Acquisition.lvclass">)  [unwired: 7 in]
              n1452 = call "Read connection.vi"("error in (no error)"=w3987, "Server in"=w3988) -> ("error out"=w3985:errorcluster, "connection"=w3986:bool, "Server out"=w3984:refnum<class "Acquisition.lvclass">)  [unwired: 7 in]
              n1453 = And(x=w3986, y=w3977) -> (x .and. y?=w3981:bool)
              n1454 = case shown="False" w3981 {
                tunnel: w3985 -> [w4040 w4057]
                tunnel: [w4040 w4056] -> w4022
                tunnel: w3984 -> [w4041 w4047]
                tunnel: [w4041 w4045] -> w4018
                tunnel: [w4036 0] -> w3973
                tunnel: w3977 -> [w4037 _]
                frame False {
                  n1455 = Select(t=8, s=w4037, f=0) -> (s? t:f=w4036:i32)
                }
                frame True {
                  n1456 = call-dynamic "Read Channel.vi"("error in (no error)"=w4057, "Acquisition in"=w4047) -> ("error out"=w4052:errorcluster, "Channel.lvclass"=w4051:refnum<class "Channel.lvclass">, "Acquisition out"=w4046:refnum<class "Acquisition.lvclass">)  [unwired: 7 in]
                  n1457 = call-dynamic "Read State Machine.vi"("error in (no error)"=w4052, "Device in"=w4051) -> ("error out"=w4053:errorcluster, "State Machine.lvclass"=w4055:refnum<class "State Machine.lvclass">, "Device out"=w4049:refnum<class "Channel.lvclass">)  [unwired: 7 in]
                  n1458 = call "Next State.vi"("error in (no error)"=w4053, "New_State"=50, "State Machine in"=w4055) -> ("error out"=w4043:errorcluster, "State Machine out"=w4044:refnum<class "State Machine.lvclass">)  [unwired: 7 in]
                  n1459 = call-dynamic "Write State Machine.vi"("error in (no error)"=w4043, "State Machine.lvclass"=w4044, "Device in"=w4049) -> ("error out"=w4048:errorcluster, "Device out"=w4050:refnum<class "Channel.lvclass">)  [unwired: 7 in]
                  n1460 = call-dynamic "Write Channel.vi"("error in (no error)"=w4048, "Channel.lvclass"=w4050, "Acquisition in"=w4046) -> ("error out"=w4056:errorcluster, "Acquisition out"=w4045:refnum<class "Acquisition.lvclass">)  [unwired: 7 in]
                }
              }
              n1461 = call-dynamic "Write AcquisitionD.vi"("error in (no error)"=w4022, "Acquisition.lvclass"=w4018, "S4ACS_GUI in"=w4019) -> ("error out"=w4012:errorcluster, "S4ACS_GUI out"=w4013:refnum<class "S4GUI.lvclass">)  [unwired: 7 in]
            }
          }
          n1462 = Compound Arithmetic op=ADD(w3893, w3892, w3891, w3890) -> (w3889:i32)
          n1463 = case shown="0, Default" w3889 {
            tunnel: w3888 -> [w3904 _ _ _ _ _ _ _ _ _ _ _ _ _ _ _]
            tunnel: [w3903 u32 1 ("Obs_state") u32 1 ("Obs_state") u32 1 ("Obs_state") u32 1 ("Obs_state") u32 1 ("Obs_state") u32 1 ("Obs_state") u32 1 ("Obs_state") u32 1 ("Obs_state") u32 1 ("Obs_state") u32 1 ("Obs_state") u32 1 ("Obs_state") u32 1 ("Obs_state") u32 1 ("Obs_state") u32 1 ("Obs_state") u32 1 ("Obs_state")] -> w3887
            tunnel: ["" ("Error Msg") "ERROR: Lost channel 1 connection... - HandleObservationSync.vi state 325" ("Error Msg") "ERROR: Lost channel 2 connection...- HandleObservationSync.vi state 325" ("Error Msg") "ERROR: Lost channels 1 and 2 connection...- HandleObservationSync.vi state 325" ("Error Msg") "ERROR: Lost channel 3 connection...- HandleObservationSync.vi state 325" ("Error Msg") "ERROR: Lost channels 1 and  3 connection...- HandleObservationSync.vi state 325" ("Error Msg") "ERROR:  Lost channels 2 and  3 connection...- HandleObservationSync.vi state 325" ("Error Msg") "ERROR:  Lost channels 1, 2 and  3 connection...- HandleObservationSync.vi state 325" ("Error Msg") "ERROR: Lost channel 4 connection...- HandleObservationSync.vi state 325" ("Error Msg") "ERROR:  Lost channels 1 and 4 connection...- HandleObservationSync.vi state 325" ("Error Msg") "ERROR:  Lost channels 2 and 4 connection...- HandleObservationSync.vi state 325" ("Error Msg") "ERROR: Lost channels 1, 2 and 4 connection...- HandleObservationSync.vi state 325" ("Error Msg") "ERROR: Lost channels 3 and 4 connection...- HandleObservationSync.vi state 325" ("Error Msg") "ERROR: Lost channels 1, 3 and 4 connection...- HandleObservationSync.vi state 325" ("Error Msg") "ERROR: Lost channels 2, 3 and 4 connection...- HandleObservationSync.vi state 325" ("Error Msg") "ERROR: Lost channels 1, 2, 3 and 4 connection...- HandleObservationSync.vi state 325" ("Error Msg")] -> w3886
            frame 0, Default {
              n1464 = Increment(x=w3904) -> (x+1=w3903:u32)
              n1465 = Tick Count (ms)() -> (millisecond timer value=w3901:u32)
              n1466 = local write "time1"(w3901) -> ()
            }
            frame 1 {
            }
            frame 2 {
            }
            frame 3 {
            }
            frame 4 {
            }
            frame 5 {
            }
            frame 6 {
            }
            frame 7 {
            }
            frame 8 {
            }
            frame 9 {
            }
            frame 10 {
            }
            frame 11 {
            }
            frame 12 {
            }
            frame 13 {
            }
            frame 14 {
            }
            frame 15 {
            }
          }
          n1467 = Bundle By Name(cluster=w3898, "Obs_state"=w3887, "Error Msg"=w3886) -> (w3897:refnum<class "S4GUI.lvclass">)
        }
        frame 326 {
          # "Espera terminar a execução do comando atual \nantes de ir ao proximo passo da Observação."
          n1468 = call-dynamic "Read AcquisitionA.vi"("error in (no error)"=w4177, "S4ACS_GUI in"=w4178) -> ("error out"=w4159:errorcluster, "Acquisition.lvclass"=w4160:refnum<class "Acquisition.lvclass">, "S4ACS_GUI out"=w4180:refnum<class "S4GUI.lvclass">)  [unwired: 7 in]
          n1469 = call "Read connection.vi"("error in (no error)"=w4159, "Server in"=w4160) -> ("error out"=w4158:errorcluster, "connection"=w4157:bool, "Server out"=w4156:refnum<class "Acquisition.lvclass">)  [unwired: 7 in]
          n1470 = case shown="False" w4157 {
            tunnel: w4158 -> [w4279 w4300]
            tunnel: [w4280 w4298] -> w4181
            tunnel: [w4279 w4297] -> w4179
            tunnel: [TRUE w4286] -> w4138
            tunnel: w4156 -> [w4280 w4289]
            tunnel: [FALSE w4281] -> w4136
            frame False {
            }
            frame True {
              n1471 = call-dynamic "Read Channel.vi"("error in (no error)"=w4300, "Acquisition in"=w4289) -> ("error out"=w4283:errorcluster, "Channel.lvclass"=w4285:refnum<class "Channel.lvclass">, "Acquisition out"=w4299:refnum<class "Acquisition.lvclass">)  [unwired: 7 in]
              n1472 = call-dynamic "Read wait_expose.vi"("error in (no error)"=w4283, "Channel in"=w4285) -> ("error out"=w4282:errorcluster, "wait_expose"=w4281:bool, "Channel out"=w4284:refnum<class "Channel.lvclass">)  [unwired: 7 in]
              n1473 = call-dynamic "Read State Machine.vi"("error in (no error)"=w4282, "Device in"=w4284) -> ("error out"=w4291:errorcluster, "State Machine.lvclass"=w4293:refnum<class "State Machine.lvclass">, "Device out"=w4295:refnum<class "Channel.lvclass">)  [unwired: 7 in]
              n1474 = call-dynamic "Read State.vi"("error in (no error)"=w4291, "State Machine in"=w4293) -> ("error out"=w4290:errorcluster, "State"=w4287:i32, "State Machine out"=w4292:refnum<class "State Machine.lvclass">)  [unwired: 7 in]
              n1475 = Greater?(x=w4287, y=53 ("x")) -> (0:w4286:bool)
              n1476 = call-dynamic "Write State Machine.vi"("error in (no error)"=w4290, "State Machine.lvclass"=w4292, "Device in"=w4295) -> ("error out"=w4294:errorcluster, "Device out"=w4296:refnum<class "Channel.lvclass">)  [unwired: 7 in]
              n1477 = call-dynamic "Write Channel.vi"("error in (no error)"=w4294, "Channel.lvclass"=w4296, "Acquisition in"=w4299) -> ("error out"=w4297:errorcluster, "Acquisition out"=w4298:refnum<class "Acquisition.lvclass">)  [unwired: 7 in]
            }
          }
          n1478 = call-dynamic "Write AcquisitionA.vi"("error in (no error)"=w4179, "Acquisition.lvclass"=w4181, "S4ACS_GUI in"=w4180) -> ("error out"=w4174:errorcluster, "S4ACS_GUI out"=w4173:refnum<class "S4GUI.lvclass">)  [unwired: 7 in]
          n1479 = call "Read AcquisitionB.vi"("error in (no error)"=w4174, "S4ACS_GUI in"=w4173) -> ("error out"=w4151:errorcluster, "Acquisition.lvclass"=w4155:refnum<class "Acquisition.lvclass">, "S4ACS_GUI out"=w4175:refnum<class "S4GUI.lvclass">)  [unwired: 7 in]
          n1480 = call "Read connection.vi"("error in (no error)"=w4151, "Server in"=w4155) -> ("error out"=w4152:errorcluster, "connection"=w4153:bool, "Server out"=w4154:refnum<class "Acquisition.lvclass">)  [unwired: 7 in]
          n1481 = case shown="True" w4153 {
            tunnel: w4152 -> [w4255 w4268]
            tunnel: w4154 -> [w4256 w4267]
            tunnel: [TRUE w4262] -> w4140
            tunnel: [w4255 w4266] -> w4172
            tunnel: [w4256 w4265] -> w4171
            tunnel: [FALSE w4257] -> w4135
            frame False {
            }
            frame True {
              n1482 = call-dynamic "Read Channel.vi"("error in (no error)"=w4268, "Acquisition in"=w4267) -> ("error out"=w4259:errorcluster, "Channel.lvclass"=w4261:refnum<class "Channel.lvclass">, "Acquisition out"=w4269:refnum<class "Acquisition.lvclass">)  [unwired: 7 in]
              n1483 = call-dynamic "Read wait_expose.vi"("error in (no error)"=w4259, "Channel in"=w4261) -> ("error out"=w4258:errorcluster, "wait_expose"=w4257:bool, "Channel out"=w4260:refnum<class "Channel.lvclass">)  [unwired: 7 in]
              n1484 = call-dynamic "Read State Machine.vi"("error in (no error)"=w4258, "Device in"=w4260) -> ("error out"=w4275:errorcluster, "State Machine.lvclass"=w4273:refnum<class "State Machine.lvclass">, "Device out"=w4271:refnum<class "Channel.lvclass">)  [unwired: 7 in]
              n1485 = call-dynamic "Read State.vi"("error in (no error)"=w4275, "State Machine in"=w4273) -> ("error out"=w4276:errorcluster, "State"=w4264:i32, "State Machine out"=w4274:refnum<class "State Machine.lvclass">)  [unwired: 7 in]
              n1486 = Greater?(x=w4264, y=53 ("x")) -> (0:w4262:bool)
              n1487 = call-dynamic "Write State Machine.vi"("error in (no error)"=w4276, "State Machine.lvclass"=w4274, "Device in"=w4271) -> ("error out"=w4272:errorcluster, "Device out"=w4270:refnum<class "Channel.lvclass">)  [unwired: 7 in]
              n1488 = call-dynamic "Write Channel.vi"("error in (no error)"=w4272, "Channel.lvclass"=w4270, "Acquisition in"=w4269) -> ("error out"=w4266:errorcluster, "Acquisition out"=w4265:refnum<class "Acquisition.lvclass">)  [unwired: 7 in]
            }
          }
          n1489 = call "Write AcquisitionB.vi"("error in (no error)"=w4172, "Acquisition.lvclass"=w4171, "S4ACS_GUI in"=w4175) -> ("error out"=w4164:errorcluster, "S4ACS_GUI out"=w4163:refnum<class "S4GUI.lvclass">)  [unwired: 7 in]
          n1490 = call-dynamic "Read AcquisitionC.vi"("error in (no error)"=w4164, "S4ACS_GUI in"=w4163) -> ("error out"=w4147:errorcluster, "Acquisition.lvclass"=w4150:refnum<class "Acquisition.lvclass">, "S4ACS_GUI out"=w4166:refnum<class "S4GUI.lvclass">)  [unwired: 7 in]
          n1491 = call "Read connection.vi"("error in (no error)"=w4147, "Server in"=w4150) -> ("error out"=w4146:errorcluster, "connection"=w4148:bool, "Server out"=w4149:refnum<class "Acquisition.lvclass">)  [unwired: 7 in]
          n1492 = case shown="True" w4148 {
            tunnel: [w4231 w4245] -> w4167
            tunnel: [w4232 w4244] -> w4165
            tunnel: w4146 -> [w4231 w4241]
            tunnel: w4149 -> [w4232 w4242]
            tunnel: [TRUE w4238] -> w4139
            tunnel: [FALSE w4233] -> w4134
            frame False {
            }
            frame True {
              n1493 = call-dynamic "Read Channel.vi"("error in (no error)"=w4241, "Acquisition in"=w4242) -> ("error out"=w4235:errorcluster, "Channel.lvclass"=w4237:refnum<class "Channel.lvclass">, "Acquisition out"=w4243:refnum<class "Acquisition.lvclass">)  [unwired: 7 in]
              n1494 = call-dynamic "Read wait_expose.vi"("error in (no error)"=w4235, "Channel in"=w4237) -> ("error out"=w4234:errorcluster, "wait_expose"=w4233:bool, "Channel out"=w4236:refnum<class "Channel.lvclass">)  [unwired: 7 in]
              n1495 = call-dynamic "Read State Machine.vi"("error in (no error)"=w4234, "Device in"=w4236) -> ("error out"=w4251:errorcluster, "State Machine.lvclass"=w4249:refnum<class "State Machine.lvclass">, "Device out"=w4247:refnum<class "Channel.lvclass">)  [unwired: 7 in]
              n1496 = call-dynamic "Read State.vi"("error in (no error)"=w4251, "State Machine in"=w4249) -> ("error out"=w4252:errorcluster, "State"=w4239:i32, "State Machine out"=w4250:refnum<class "State Machine.lvclass">)  [unwired: 7 in]
              n1497 = Greater?(x=w4239, y=53 ("x")) -> (0:w4238:bool)
              n1498 = call-dynamic "Write State Machine.vi"("error in (no error)"=w4252, "State Machine.lvclass"=w4250, "Device in"=w4247) -> ("error out"=w4248:errorcluster, "Device out"=w4246:refnum<class "Channel.lvclass">)  [unwired: 7 in]
              n1499 = call-dynamic "Write Channel.vi"("error in (no error)"=w4248, "Channel.lvclass"=w4246, "Acquisition in"=w4243) -> ("error out"=w4245:errorcluster, "Acquisition out"=w4244:refnum<class "Acquisition.lvclass">)  [unwired: 7 in]
            }
          }
          n1500 = call-dynamic "Write AcquisitionC.vi"("error in (no error)"=w4167, "Acquisition.lvclass"=w4165, "S4ACS_GUI in"=w4166) -> ("error out"=w4161:errorcluster, "S4ACS_GUI out"=w4162:refnum<class "S4GUI.lvclass">)  [unwired: 7 in]
          n1501 = call-dynamic "Read AcquisitionD.vi"("error in (no error)"=w4161, "S4ACS_GUI in"=w4162) -> ("error out"=w4142:errorcluster, "Acquisition.lvclass"=w4145:refnum<class "Acquisition.lvclass">, "S4ACS_GUI out"=w4168:refnum<class "S4GUI.lvclass">)  [unwired: 7 in]
          n1502 = call "Read connection.vi"("error in (no error)"=w4142, "Server in"=w4145) -> ("error out"=w4141:errorcluster, "connection"=w4143:bool, "Server out"=w4144:refnum<class "Acquisition.lvclass">)  [unwired: 7 in]
          n1503 = case shown="True" w4143 {
            tunnel: [w4208 w4228] -> w4170
            tunnel: [w4207 w4227] -> w4169
            tunnel: w4144 -> [w4208 w4226]
            tunnel: w4141 -> [w4207 w4225]
            tunnel: [TRUE w4214] -> w4137
            tunnel: [FALSE w4209] -> w4133
            frame False {
            }
            frame True {
              n1504 = call-dynamic "Read Channel.vi"("error in (no error)"=w4225, "Acquisition in"=w4226) -> ("error out"=w4211:errorcluster, "Channel.lvclass"=w4213:refnum<class "Channel.lvclass">, "Acquisition out"=w4224:refnum<class "Acquisition.lvclass">)  [unwired: 7 in]
              n1505 = call-dynamic "Read wait_expose.vi"("error in (no error)"=w4211, "Channel in"=w4213) -> ("error out"=w4210:errorcluster, "wait_expose"=w4209:bool, "Channel out"=w4212:refnum<class "Channel.lvclass">)  [unwired: 7 in]
              n1506 = call-dynamic "Read State Machine.vi"("error in (no error)"=w4210, "Device in"=w4212) -> ("error out"=w4218:errorcluster, "State Machine.lvclass"=w4220:refnum<class "State Machine.lvclass">, "Device out"=w4222:refnum<class "Channel.lvclass">)  [unwired: 7 in]
              n1507 = call-dynamic "Read State.vi"("error in (no error)"=w4218, "State Machine in"=w4220) -> ("error out"=w4217:errorcluster, "State"=w4215:i32, "State Machine out"=w4219:refnum<class "State Machine.lvclass">)  [unwired: 7 in]
              n1508 = Greater?(x=w4215, y=53 ("x")) -> (0:w4214:bool)
              n1509 = call-dynamic "Write State Machine.vi"("error in (no error)"=w4217, "State Machine.lvclass"=w4219, "Device in"=w4222) -> ("error out"=w4221:errorcluster, "Device out"=w4223:refnum<class "Channel.lvclass">)  [unwired: 7 in]
              n1510 = call-dynamic "Write Channel.vi"("error in (no error)"=w4221, "Channel.lvclass"=w4223, "Acquisition in"=w4224) -> ("error out"=w4227:errorcluster, "Acquisition out"=w4228:refnum<class "Acquisition.lvclass">)  [unwired: 7 in]
            }
          }
          n1511 = call-dynamic "Write AcquisitionD.vi"("error in (no error)"=w4169, "Acquisition.lvclass"=w4170, "S4ACS_GUI in"=w4168) -> ("error out"=w4126:errorcluster, "S4ACS_GUI out"=w4128:refnum<class "S4GUI.lvclass">)  [unwired: 7 in]
          n1512 = Compound Arithmetic op=AND(w4138, w4140, w4139, w4137) -> (w4131:bool)
          n1513 = Compound Arithmetic op=OR(w4136, w4135, w4134, w4133) -> (w4132:bool)
          n1514 = call-dynamic "VerifErrors.vi"("error in (no error)"=w4126, "S4GUI in"=w4128) -> ("error out"=w4125:errorcluster, "Error value"=w4124:u32, "S4GUI out"=w4127:refnum<class "S4GUI.lvclass">)  [unwired: 7 in]
          n1515 = case shown="False" w4131 {
            tunnel: w4127 -> [w4185 w4204]
            tunnel: [w4183 w4203] -> w4129
